vi "FTW-Ether-NewLoggerConnection.vi"(5 "Logger Address":string, 11 "error in":errorcluster) -> (4 "Event Logger Connection":refnum<class "FTW-Logger.lvclass">, 15 "error out":errorcluster)   [LabVIEW 2012, in "FTW-Actor.lvlib" / "FTW-Ether.lvclass"]
uses:
  FTW-Ether.lvclass
  EventLogger/FTW-Logger.lvclass
  FTW-Ether-Instance.vi
panel:
  # "Inputs"
  # "Outputs"
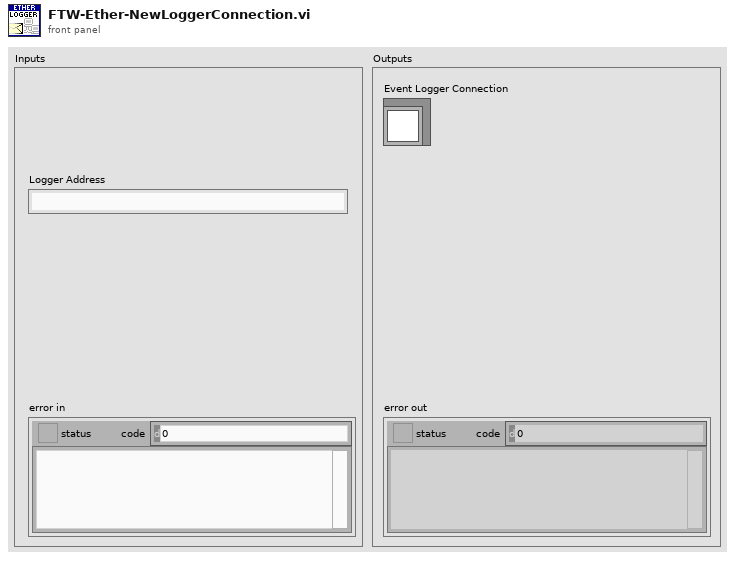
[diagram p1: front panel]
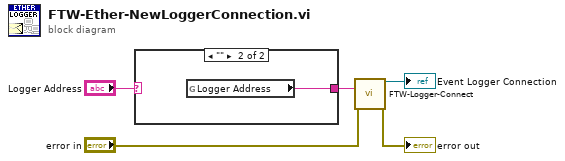
[diagram p0: block diagram]
diagram:
  n1 = case shown="\"\"" "Logger Address" {
    selector: "Logger Address" -> [w6 _]
    tunnel: [w6 w7] -> w2
    frame Default {
    }
    frame "" {
      n2 = global read "FTW-Ether-Instance.vi" "Logger Address"() -> (w7:string)
    }
  }
  n3 = call "FTW-Logger-Connect.vi"("Logger Address"=w2, "error in"="error in") -> ("FTW Logger Connector"=→"Event Logger Connection":refnum<class "FTW-Logger.lvclass">, "error out"=→"error out":errorcluster)  [unwired: 12 in]
